vi "CollectImageSet (SubVI).vi"(8 "error in":errorcluster, 9 "Axes Speeds [mm/s]":T4={"X Speed"=10.0, "Y Speed"=10.0, "Z Speed"=10.0}, 10 "Set of Coordinates to Process":dbl[][](array[numeric]), 11 "Session in":T1) -> (0 "error out":errorcluster, 1 "Image Array":T2[](array[plugin-control])=["image_0", "image_1", "image_2", "image_3", "image_4", "image_5", "image_6", "image_7", "image_8", "image_9", "image_10", "image_11", "image_12", "image_13", "image_14", "image_15", "image_16", "image_17", "image_18", "image_19", "image_20", "image_21", "image_22", "image_23", "image_24", "image_25", "image_26", "image_27", "image_28", "image_29", "image_30", "image_31", "image_32", "image_33", "image_34", "image_35", "image_36", "image_37", "image_38", "image_39", "image_40", "image_41", "image_42", "image_43", "image_44", "image_45", "image_46", "image_47", "image_48", "image_49", "image_50", "image_51", "image_52", "image_53", "image_54", "image_55", "image_56", "image_57", "image_58", "image_59", "image_60", "image_61", "image_62", "image_63", "image_64", "image_65", "image_66", "image_67", "image_68", "image_69", "image_70", "image_71", "image_72", "image_73", "image_74", "image_75", "image_76", "image_77", "image_78", "image_79"], 2 "Captured positions":dbl[][](array[numeric]), 3 "Session out":T1, 5 "Moving":bool, 7 "XYZ Stage Current Position":T3)   [LabVIEW 2016]
uses:
  <vilib>/userdefined/High Color/IMAQdx.ctl
  <vilib>/vision/driver/NI_Vision_Acquisition_Software.lvlib
  <vilib>/vision/NI_Vision_Development_Module.lvlib
panel:
  out "Most recently collected image":T2(plugin-control)
  out "Image #":i32
  out "Finished!":bool
  out "Object Location [mm]":T5
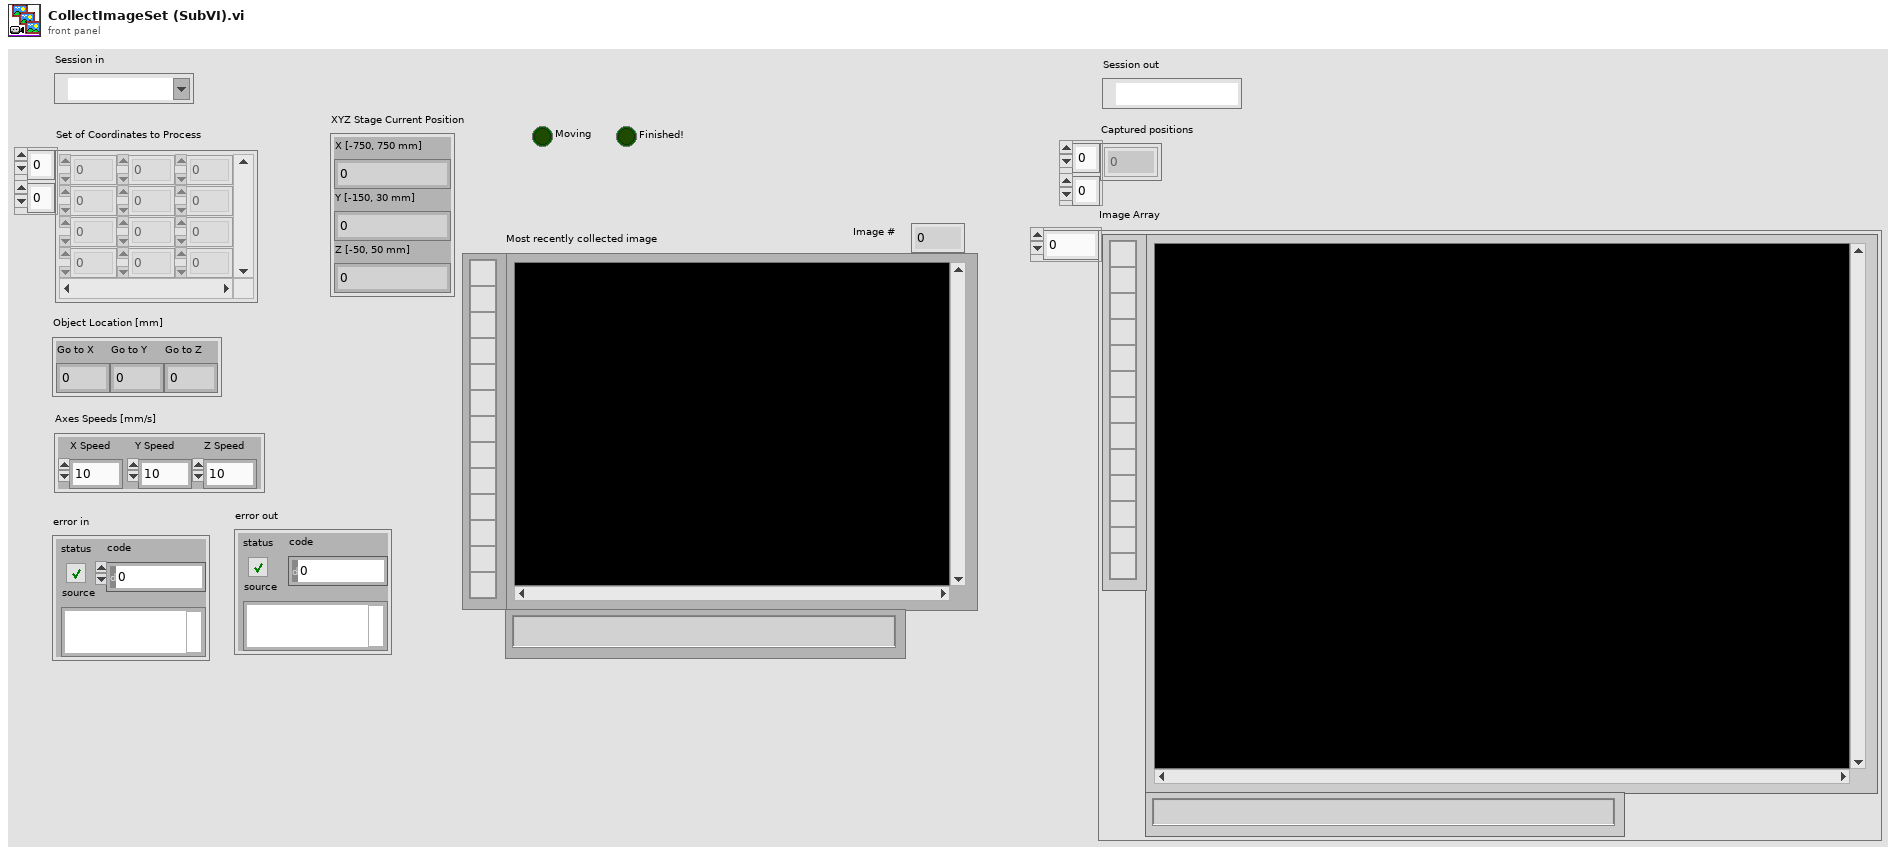
[diagram p1: front panel]
types:
  T1 = typedef "IMAQdx.ctl" = refnum<k21>
  T2 = typedef "IMAQ Image.ctl" = refnum<image>
  T3 = cluster{"X [-750, 750 mm]":dbl, "Y [-150, 30 mm]":dbl, "Z [-50, 50 mm]":dbl}
  T4 = cluster{"X Speed":dbl, "Y Speed":dbl, "Z Speed":dbl}
  T5 = cluster{"Go to X":dbl, "Go to Y":dbl, "Go to Z":dbl}
  T6 = cluster{"Set of Coordinates to Process[0]":dbl, "Set of Coordinates to Process[1]":dbl, "Set of Coordinates to Process[2]":dbl}
  T7 = typedef "Image Type" = u32
  T8 = cluster{"Final X":dbl, "Final Y":dbl, "Final Z":dbl}
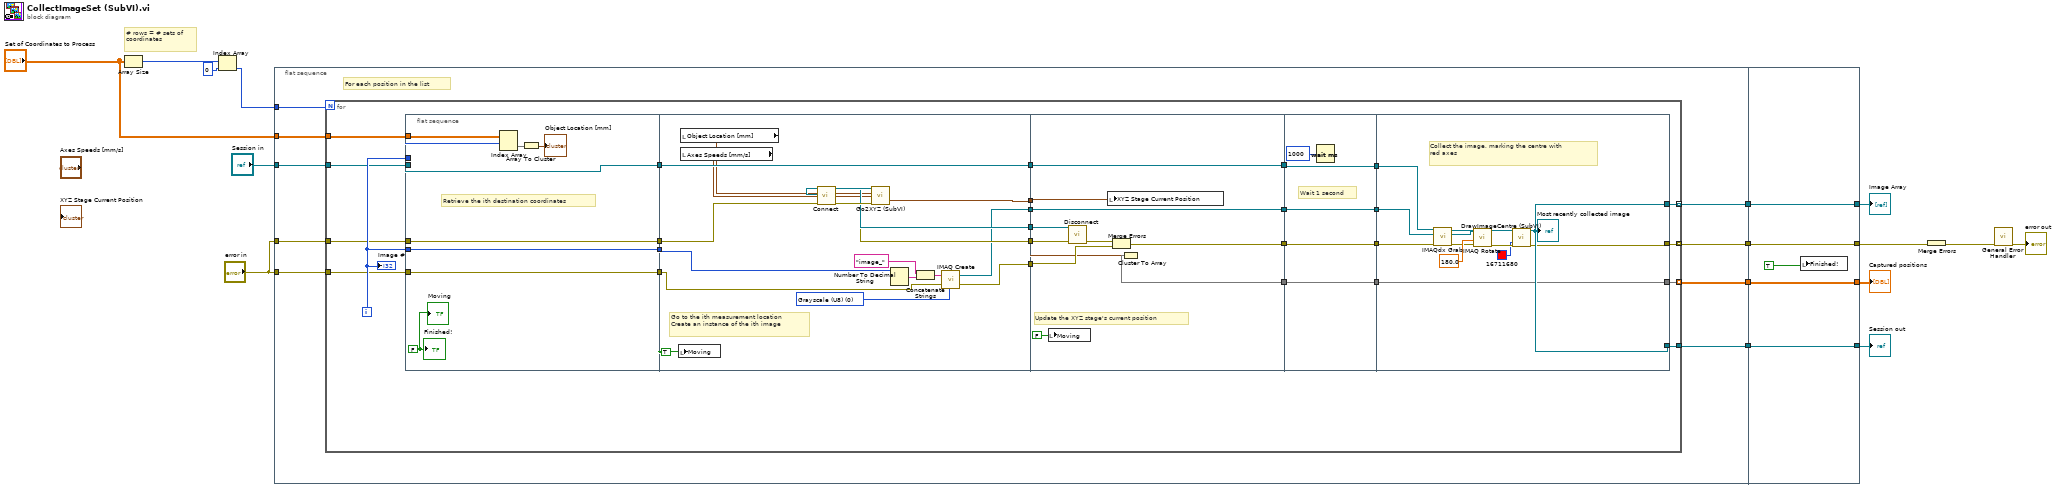
[diagram p0: block diagram]
diagram:
  # "# rows = # sets of\ncoordinates"
  n1 = Array Size(array="Set of Coordinates to Process") -> (size(s)=w4:i32[])
  n2 = Index Array(array=w4, index=0) -> (element=w6:i32)
  n3 = flat-sequence {
    tunnel: w6 -> [w25]
    tunnel: "Session in" -> [w24]
    tunnel: "error in" -> [w20]
    tunnel: "error in" -> [w18]
    tunnel: [w23] -> w16
    tunnel: [w22] -> w15
    tunnel: [w21] -> w14
    tunnel: [w19] -> w13
    tunnel: "Set of Coordinates to Process" -> [w17]
    tunnel: [w109] -> w11
    tunnel: [w110] -> w10
    tunnel: [w111] -> w9
    tunnel: [w112] -> w8
    tunnel: w16 -> [w112]
    tunnel: w15 -> [w111]
    tunnel: w14 -> [w110]
    tunnel: w13 -> [w109]
    frame #0 {
      # "For each position in the list"
      n4 = for {
        N: w25 -> [_]
        tunnel: w24 -> [w40]
        tunnel: [w39] -> w23 mode=indexing
        tunnel: w20 -> [w37]
        tunnel: w18 -> [w35]
        tunnel: [w31] -> w22
        tunnel: [w30] -> w19 mode=indexing
        tunnel: [w27] -> w21 mode=indexing
        tunnel: w17 -> [w26]
        i -> [w48]
        n5 = flat-sequence {
          tunnel: w48 -> [w61]
          tunnel: w48 -> [w60]
          tunnel: [w60] -> w49
          tunnel: [w59] -> w41
          tunnel: w40 -> [w59]
          tunnel: [w58] -> w38
          tunnel: w37 -> [w58]
          tunnel: [w57] -> w36
          tunnel: w35 -> [w57]
          tunnel: w26 -> [w56]
          tunnel: [w76] -> w52
          tunnel: [w75] -> w51
          tunnel: [w74] -> w50
          tunnel: w49 -> [w69]
          tunnel: [w71] -> w45
          tunnel: [w70] -> w42
          tunnel: w41 -> [w70]
          tunnel: w38 -> [w67]
          tunnel: w36 -> [w62]
          tunnel: [w66] -> w32
          tunnel: w52 -> [w89]
          tunnel: w51 -> [w81]
          tunnel: w50 -> [w88]
          tunnel: [w87] -> w46
          tunnel: w45 -> [w87]
          tunnel: [w86] -> w43
          tunnel: w42 -> [w86]
          tunnel: [w83] -> w33
          tunnel: w32 -> [w84]
          tunnel: [w82] -> w29
          tunnel: [w93] -> w47
          tunnel: w46 -> [w93]
          tunnel: [w92] -> w44
          tunnel: w43 -> [w92]
          tunnel: [w91] -> w34
          tunnel: w33 -> [w91]
          tunnel: w29 -> [w90]
          tunnel: [w90] -> w28
          tunnel: w47 -> [w107]
          tunnel: w44 -> [w106]
          tunnel: [w96] -> w39
          tunnel: w34 -> [w103]
          tunnel: [w101] -> w31
          tunnel: [w97] -> w30
          tunnel: w28 -> [w100]
          tunnel: [w100] -> w27
          frame #0 {
            w53 = FALSE ("Finished!")
            # "Retrieve the ith destination coordinates"
            n6 = Index Array(array=w56, index (row)=w61) -> (element=w55:dbl[])  [unwired: 1 in]
            n7 = Array To Cluster(array=w55) -> (cluster=→"Object Location [mm]":T6)
            "Finished!" <- w53
            "Moving" <- w53
          }
          frame #1 {
            w79 = T7 0 items=["Grayscale (U8)", "Grayscale (I16)", "Grayscale (SGL)", "Complex (CSG)", "RGB (U32)", "HSL (U32)", "RGB (U64)", "Grayscale (U16)"] ("Image Type")
            # "Go to the ith measurement location\nCreate an instance of the ith image"
            n8 = local write "Moving"(TRUE ("Moving")) -> ()
            n9 = local read "Object Location [mm]"() -> (w64:T5)
            n10 = local read "Axes Speeds [mm/s]"() -> (w65:T4)
            n11 = call "Connect.vi"("error in (no error)"=w67) -> ("error out"=w77:errorcluster, "controller"=w78:refnum<k24>)  [unwired: 9 in]
            n12 = call "Go2XYZ (SubVI).vi"(".NET Refnum in"=w78, "Go to Coordinates"=w64, "Axis Speeds"=w65, "error in (no error)"=w77) -> (".NET Refnum out"=w76:refnum<k24>, "Final Position"=w75:T8, "error out"=w74:errorcluster)  [unwired: 8 in, 1 out]
            n13 = Number To Decimal String(number=w69) -> (decimal integer string=w68:string)  [unwired: 1 in]
            n14 = Concatenate Strings("image_" ("Image Name"), w68) -> (w72:string)
            n15 = call "IMAQ Create"("Image Name"=w72, "Image Type"=w79, "error in (no error)"=w62) -> ("New Image"=w71:T2, "error out"=w66:errorcluster)  [unwired: 1 in, 1 out]
          }
          frame #2 {
            # "Update the XYZ stage's current position"
            n16 = local write "Moving"(FALSE ("Moving")) -> ()
            n17 = call "Disconnect.vi"("error in (no error)"=w88, "controller"=w89) -> ("error out"=w85:errorcluster)  [unwired: 9 in]
            n18 = local write "XYZ Stage Current Position"(w81) -> ()
            n19 = Merge Errors(w85, w84) -> (w83:errorcluster)
            n20 = Cluster To Array(cluster=w81) -> (array=w82:dbl[])
          }
          frame #3 {
            # "Wait 1 second"
            n21 = Wait (ms)(milliseconds to wait=u32 1000) -> ()  [unwired: 1 out]
          }
          frame #4 {
            # "Collect the image, marking the centre with \nred axes"
            n22 = call <vilib>:"IMAQdx Grab.vi"("error in"=w103, "Image In"=w107, "Session In"=w106) -> ("error out"=w102:errorcluster, "Image Out"=w105:T2, "Session Out"=w101:T1)  [unwired: 1 in, 5 out]
            n23 = call "IMAQ Rotate"("error in (no error)"=w102, "Angle (degrees)"=sgl 180.0, "Image Src"=w105) -> ("error out"=w98:errorcluster, "Image Dst Out"=w99:T2)  [unwired: 7 in]
            n24 = call "DrawImageCentre (SubVI).vi"("Axis colour"=u32 16711680, "error in (no error)"=w98, "Refnum in"=w99) -> ("error out"=w97:errorcluster, "Refnum out"=w96:T2)  [unwired: 7 in]
            "Most recently collected image" <- w96
          }
        }
        "Image #" <- w48
      }
    }
    frame #1 {
      n25 = local write "Finished!"(TRUE ("Finished!")) -> ()
    }
  }
  n26 = Merge Errors(w11) -> (w12:errorcluster)
  n27 = call <vilib>:"General Error Handler.vi"("error in (no error)"=w12) -> ("error out"=→"error out":errorcluster)  [unwired: 2 in, 12 out]
  "Image Array" <- w8
  "Captured positions" <- w10
  "Session out" <- w9
